vi "getRowElements.vi"(8 "error in (no error)":errorcluster, 11 "Goal in":refnum<class "Goal.lvclass">) -> (0 "error out":errorcluster, 2 "Row Interface":string[](array[string]), 3 "Goal out":refnum<class "Goal.lvclass">)   [LabVIEW 2020, in "Goal.lvclass"]
uses:
  Goal.lvclass
  Category/Category.lvclass
  UserEditableAmount/UserEditableAmount.lvclass
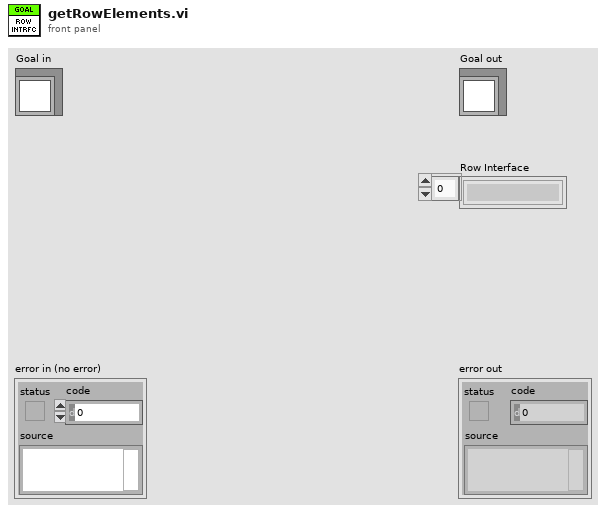
[diagram p1: front panel]
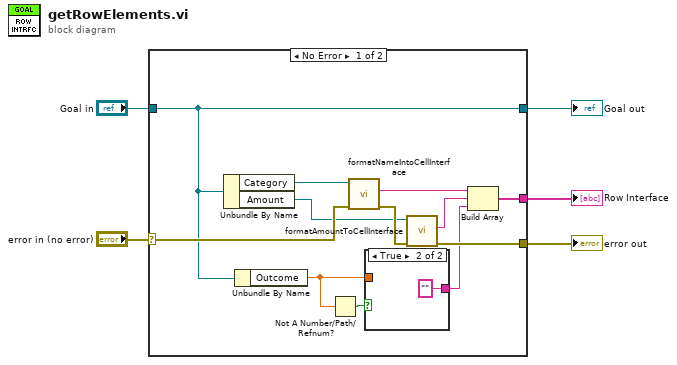
[diagram p0: block diagram]
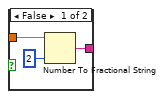
[diagram p2: hidden frame]
diagram:
  n1 = case shown="No Error" "error in (no error)" {
    selector: "error in (no error)" -> [w16 w23]
    tunnel: [w12 w23] -> w4
    tunnel: [w10 w22] -> w2
    tunnel: "Goal in" -> [w10 w22]
    tunnel: [w11 _] -> w1
    frame No Error {
      n2 = Unbundle By Name(w10) -> ("Category"=w17:refnum<class "Category.lvclass">, "Amount"=w6:refnum<class "UserEditableAmount.lvclass">)
      n3 = Unbundle By Name(w10) -> ("Outcome"=w8:dbl)
      n4 = Not A Number/Path/Refnum?(number/path/refnum=w8) -> (NaN/Path/Refnum?=w7:bool)
      n5 = call "formatNameIntoCellInterface.vi"("error in (no error)"=w16, "Category in"=w17) -> ("error out"=w15:errorcluster, "Name"=w14:string)  [unwired: 7 in, 1 out]
      n6 = case shown="True" w7 {
        tunnel: [w19 ""] -> w9
        tunnel: w8 -> [w18 _]
        frame False {
          n7 = Number To Fractional String(number=w18, precision (6)=i16 2) -> (F-format string=w19:string)  [unwired: 2 in]
        }
        frame True {
        }
      }
      n8 = call "formatAmountToCellInterface.vi"("error in (no error)"=w15, "UserEditableAmount in"=w6) -> ("error out"=w12:errorcluster, "Cell Interface"=w13:string)  [unwired: 7 in, 1 out]
      n9 = Build Array(w14, w13, w9) -> (w11:string[])
    }
    frame Error {
    }
  }
  "error out" <- w4
  "Goal out" <- w2
  "Row Interface" <- w1
